vi "Set_Initial_State.vi"(4 "SD":dbl=1.0, 5 "Tau_Off":i32, 6 "Asymmetry (X, Y)":dbl[](array[numeric]), 7 "Tau_On":i32, 11 "Ini_Anchor_Posi":dbl[][](array[numeric])) -> (0 "Center State at T":T2, 1 "Ini_Anchor_Posi":dbl[][](array[numeric]), 3 "On_Particle State":T1(array[cluster]))   [LabVIEW 2020]
uses:
  <vilib>/Analysis/baseanly.llb/Mean (DBL).vi
  <vilib>/Analysis/NI_AALBase.lvlib
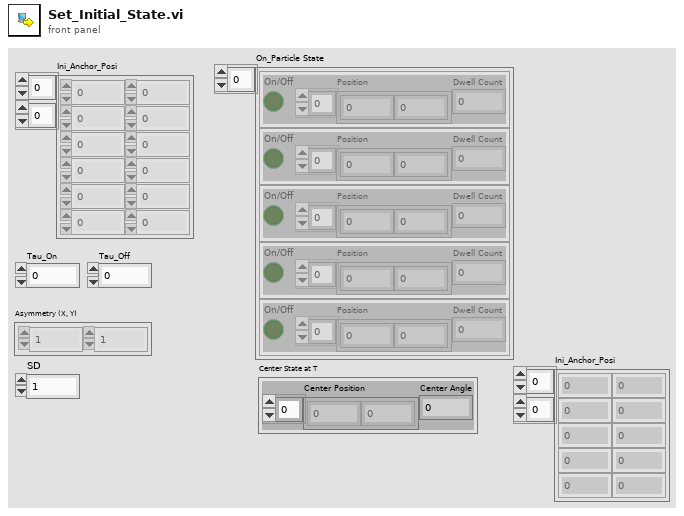
[diagram p1: front panel]
types:
  T1 = cluster{"On/Off":bool, "Position":dbl[], "Dwell Count":i32}[]
  T2 = cluster{"Center Position":dbl[], "Center Angle":dbl}
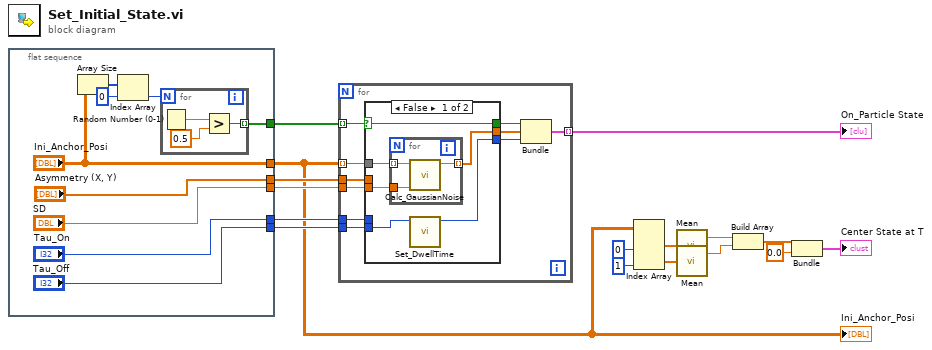
[diagram p0: block diagram]
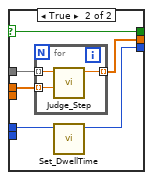
[diagram p2: hidden frame]
diagram:
  n1 = flat-sequence {
    tunnel: ["SD"] -> w14
    tunnel: ["Tau_On"] -> w16
    tunnel: ["Tau_Off"] -> w15
    tunnel: ["Asymmetry (X, Y)"] -> w13
    tunnel: ["Ini_Anchor_Posi"] -> w11
    tunnel: [w18] -> w1
    frame #0 {
      n2 = Array Size(array="Ini_Anchor_Posi") -> (size(s)=w21:i32[])
      n3 = Index Array(array=w21, index=0) -> (element=w19:i32)
      n4 = for {
        N: w19 -> [_]
        tunnel: [w26] -> w18 mode=indexing
        n5 = Random Number (0-1)() -> (number: 0 to 1=w28:dbl)
        n6 = Greater?(x=w28, y=0.5) -> (0:w26:bool)
      }
    }
  }
  n7 = for {
    tunnel: w16 -> [w38]
    tunnel: w15 -> [w37]
    tunnel: w14 -> [w36]
    tunnel: w13 -> [w35]
    tunnel: w11 -> [w31] mode=indexing
    tunnel: [w30] -> w12 mode=indexing
    tunnel: w1 -> [w29] mode=indexing
    n8 = case shown="FALSE" w29 {
      selector: w29 -> [w40 w49]
      tunnel: w38 -> [_ w53]
      tunnel: [w43 w52] -> w32
      tunnel: w37 -> [w44 _]
      tunnel: w36 -> [w42 _]
      tunnel: w31 -> [w41 w51]
      tunnel: w35 -> [_ w50]
      tunnel: [w40 w49] -> w34
      tunnel: [w39 w48] -> w33
      frame False {
        n9 = for {
          tunnel: w42 -> [w47]
          tunnel: w41 -> [w46] mode=indexing
          tunnel: [w45] -> w39 mode=indexing
          n10 = call "Calc_GaussianNoise.vi"("SD"=w47, "Start Position"=w46) -> ("Final Position"=w45:dbl)  [unwired: 9 in]
        }
        n11 = call "Set_DwellTime.vi"("Tau"=w44) -> ("Next Dwell"=w43:i32)  [unwired: 10 in]
      }
      frame True {
        n12 = for {
          tunnel: w51 -> [w56] mode=indexing
          tunnel: w50 -> [w55] mode=indexing
          tunnel: [w54] -> w48 mode=indexing
          n13 = call "Judge_Step.vi"("Asymmetry"=w55, "Position"=w56) -> ("New Position"=w54:dbl)  [unwired: 8 in, 1 out]
        }
        n14 = call "Set_DwellTime.vi"("Tau"=w53) -> ("Next Dwell"=w52:i32)  [unwired: 10 in]
      }
    }
    n15 = Bundle(w34, w33, "Next Dwell"=w32) -> (w30:cluster{bool, dbl[], "Next Dwell":i32})  [unwired: 1 in]
  }
  "On_Particle State" <- w12
  n16 = Index Array(array=w11, index (col) #1=0 ("disabled index (col)"), index (col) #2=1 ("index (col)")) -> (element #1=w7:dbl[], element #2=w8:dbl[])  [unwired: 2 in]
  n17 = call-poly <vilib>:"Mean.vi"("X"=w7) -> ("mean"=w6:dbl)  [unwired: 1 out]
  n18 = call-poly <vilib>:"Mean.vi"("X"=w8) -> ("mean"=w5:dbl)  [unwired: 1 out]
  n19 = Build Array(w6, w5) -> (w4:dbl[])
  n20 = Bundle(w4, 0.0) -> (→"Center State at T":cluster{dbl[], dbl})  [unwired: 1 in]
  "Ini_Anchor_Posi" <- w11
